vi "newLine.vi"(10 "scan info":T2, 11 "reader status in":T1) -> (3 "reader status out":T1)   [LabVIEW 2010]
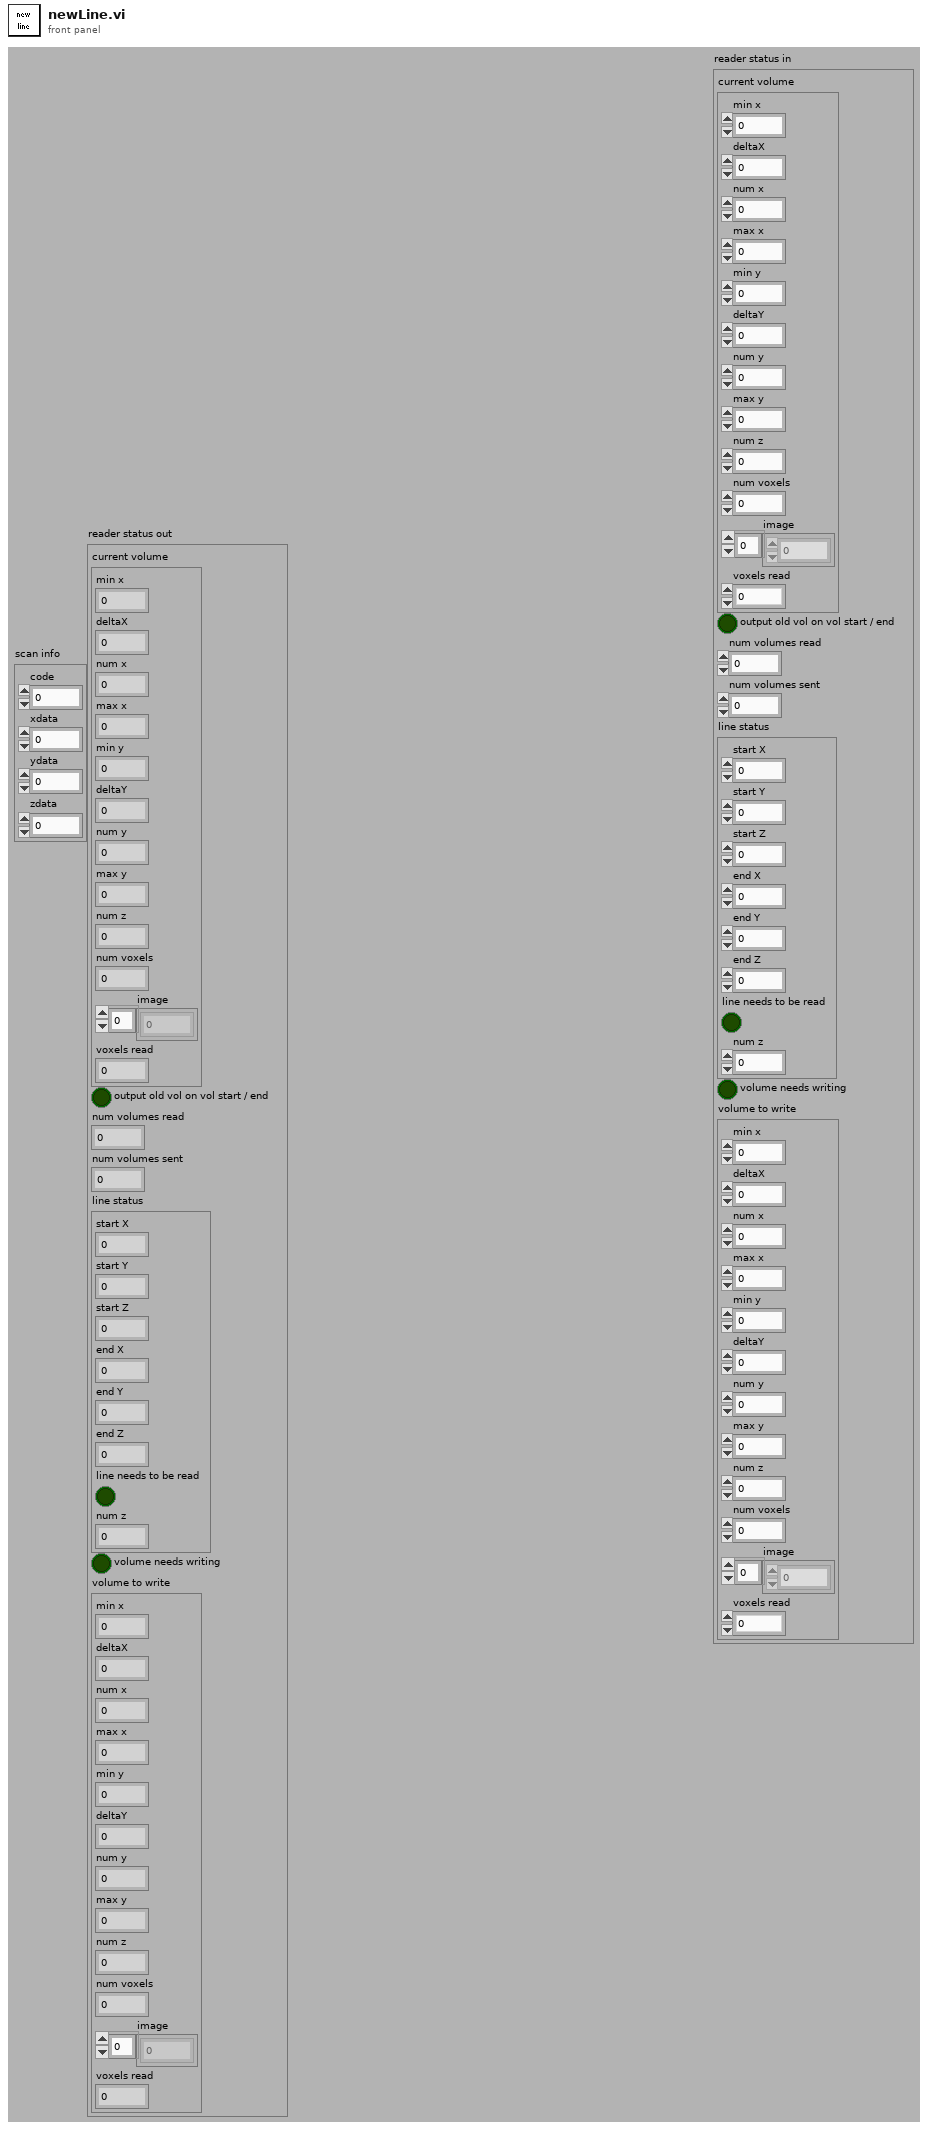
[diagram p1: front panel]
types:
  T1 = cluster{"current volume":cluster{"min x":i16, "deltaX":dbl, "num x":u32, "max x":i16, "min y":i16, "deltaY":dbl, "num y":u32, "max y":i16, "num z":u32, "num voxels":u32, "image":u32[], "voxels read":u32}, "output old vol on vol start / end":bool, "num volumes read":u32, "num volumes sent":u32, "line status":cluster{"start X":i16, "start Y":i16, "start Z":i16, "end X":i16, "end Y":i16, "end Z":i16, "line needs to be read":bool, "num z":u8}, "volume needs writing":bool, "volume to write":cluster{"min x":i16, "deltaX":dbl, "num x":u32, "max x":i16, "min y":i16, "deltaY":dbl, "num y":u32, "max y":i16, "num z":u32, "num voxels":u32, "image":u32[], "voxels read":u32}}
  T2 = cluster{"code":i32, "xdata":i32, "ydata":i32, "zdata":i32}
  T3 = enum16{"NONE", "VOLUME_START", "LINE_START", "LINE_END", "VOLUME_END"}
  T4 = cluster{"start X":i16, "start Y":i16, "start Z":i16, "end X":i16, "end Y":i16, "end Z":i16, "line needs to be read":bool, "num z":u8}
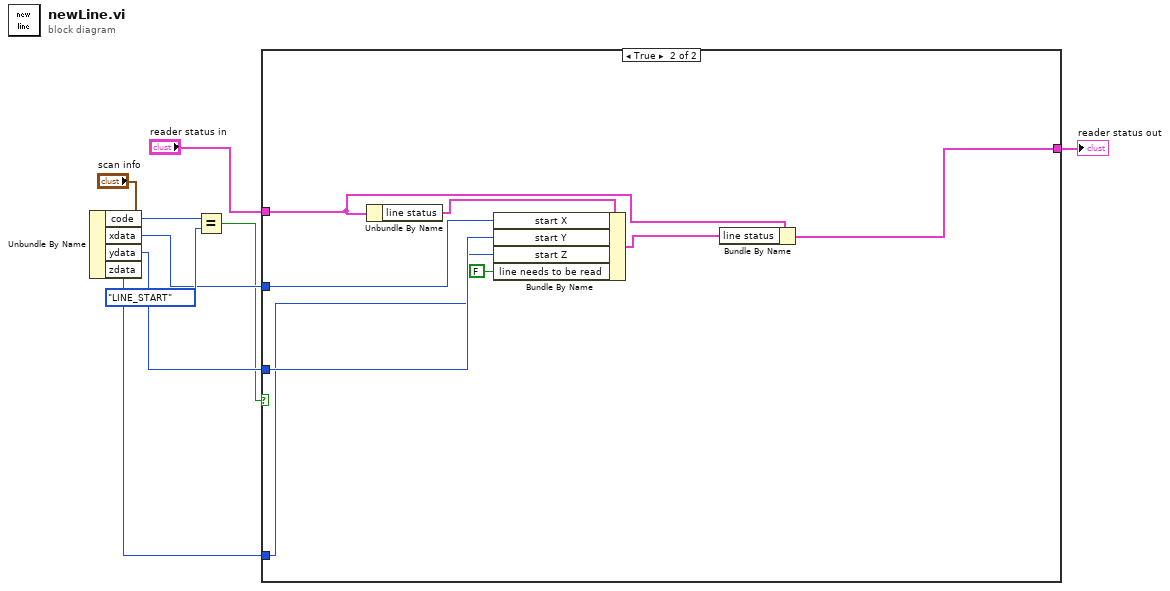
[diagram p0: block diagram]
diagram:
  n1 = Unbundle By Name("scan info") -> ("code"=w8:i32, "xdata"=w6:i32, "ydata"=w5:i32, "zdata"=w4:i32)
  n2 = Equal?(x=w8, y=T3."LINE_START" ("message")) -> (x = y?=w2:bool)
  n3 = case shown="True" w2 {
    tunnel: w6 -> [_ w17]
    tunnel: w5 -> [_ w16]
    tunnel: w4 -> [_ w15]
    tunnel: "reader status in" -> [w10 w13]
    tunnel: [w10 w11] -> w1
    frame False {
    }
    frame True {
      n4 = Unbundle By Name(w13) -> ("line status"=w18:T4)
      n5 = Bundle By Name(cluster=w18, "start X"=w17, "start Y"=w16, "start Z"=w15, "line needs to be read"=FALSE) -> (w12:T4)
      n6 = Bundle By Name(cluster=w13, "line status"=w12) -> (w11:T1)
    }
  }
  "reader status out" <- w1
